vi "动态调用VI之间的数据.vi"() -> ()   [LabVIEW 2011]
panel:
  in  "Boolean":bool
  out "error IO":errorcluster
  out "signal type":T1(ring)
  out "frequency":dbl
  out "amplitude":dbl
  out "phase":dbl
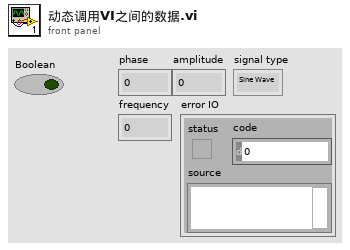
[diagram p1: front panel]
types:
  T1 = enum16{"Sine Wave", "Triangle Wave", "Square Wave", "Sawtooth Wave"}
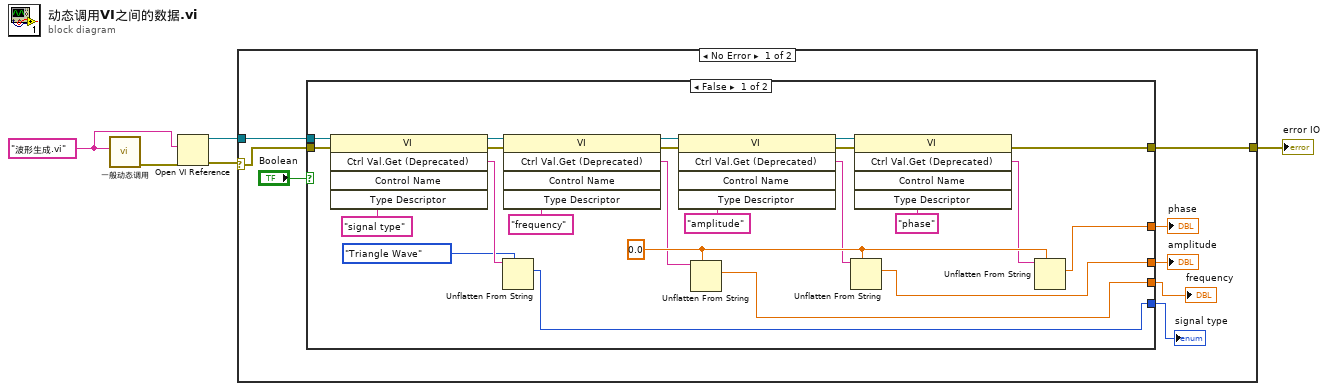
[diagram p0: block diagram]
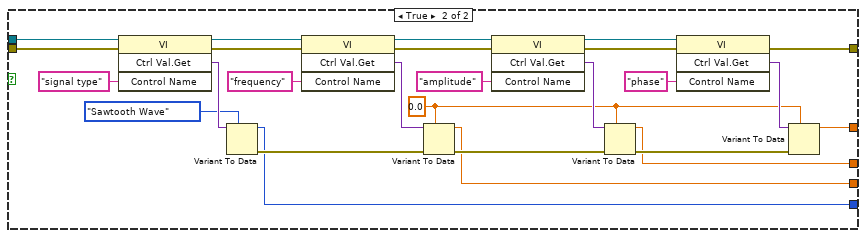
[diagram p2: hidden frame]
diagram:
  w4 = "波形生成.vi" ("name or relative path")
  n1 = call "一般动态调用.vi"("name or relative path"=w4) -> ("error out"=w5:errorcluster)  [unwired: 10 in]
  n2 = Open VI Reference(vi path=w4, error in (no error)=w5) -> (vi reference=w3:refnum<vi>, error out=w2:errorcluster)  [unwired: 4 in]
  n3 = case shown="No Error" w2 {
    selector: w2 -> [w12 w63]
    tunnel: w3 -> [w13 _]
    tunnel: [w7 w63] -> w1
    frame No Error {
      n4 = case shown="False" "Boolean" {
        tunnel: w13 -> [w36 w62]
        tunnel: w12 -> [w35 w61]
        tunnel: [w18 w41] -> w11
        tunnel: [w17 w40] -> w10
        tunnel: [w16 w39] -> w9
        tunnel: [w15 w38] -> w8
        tunnel: [w14 w37] -> w7
        frame False {
          w26 = 0.0 ("phase")
          n5 = invoke class="VI" method="Ctrl Val.Get (Deprecated)"(reference=w36, error in=w35, "Control Name"="signal type" ("控件名")) -> (reference out=w31:refnum<vi>, error out=w30:errorcluster, "Get Control Value"=w33:string)  [unwired: 2 in, 2 out]
          n6 = Unflatten From String(type=T1."Triangle Wave" ("signal type"), binary string=w33) -> (value=w15:T1)  [unwired: 3 in, 2 out]
          n7 = invoke class="VI" method="Ctrl Val.Get (Deprecated)"(reference=w31, error in=w30, "Control Name"="frequency" ("控件名")) -> (reference out=w25:refnum<vi>, error out=w24:errorcluster, "Get Control Value"=w21:string)  [unwired: 2 in, 2 out]
          n8 = invoke class="VI" method="Ctrl Val.Get (Deprecated)"(reference=w25, error in=w24, "Control Name"="amplitude" ("控件名")) -> (reference out=w23:refnum<vi>, error out=w22:errorcluster, "Get Control Value"=w20:string)  [unwired: 2 in, 2 out]
          n9 = Unflatten From String(type=w26, binary string=w21) -> (value=w16:dbl)  [unwired: 3 in, 2 out]
          n10 = Unflatten From String(type=w26, binary string=w20) -> (value=w17:dbl)  [unwired: 3 in, 2 out]
          n11 = invoke class="VI" method="Ctrl Val.Get (Deprecated)"(reference=w23, error in=w22, "Control Name"="phase" ("控件名")) -> (error out=w14:errorcluster, "Get Control Value"=w19:string)  [unwired: 2 in, 3 out]
          n12 = Unflatten From String(type=w26, binary string=w19) -> (value=w18:dbl)  [unwired: 3 in, 2 out]
        }
        frame True {
          w42 = 0.0
          n13 = invoke class="VI" method="Ctrl Val.Get"(reference=w62, error in=w61, "Control Name"="signal type") -> (reference out=w60:refnum<vi>, error out=w59:errorcluster, "Get Control Value Variant"=w58:variant)  [unwired: 1 in, 1 out]
          n14 = Variant To Data(type=T1."Sawtooth Wave", Variant=w58) -> (data=w38:T1, error out=w55:errorcluster)  [unwired: 1 in]
          n15 = invoke class="VI" method="Ctrl Val.Get"(reference=w60, error in=w59, "Control Name"="frequency") -> (reference out=w51:refnum<vi>, error out=w50:errorcluster, "Get Control Value Variant"=w54:variant)  [unwired: 1 in, 1 out]
          n16 = Variant To Data(error in=w55, type=w42, Variant=w54) -> (data=w39:dbl, error out=w48:errorcluster)
          n17 = invoke class="VI" method="Ctrl Val.Get"(reference=w51, error in=w50, "Control Name"="amplitude") -> (reference out=w47:refnum<vi>, error out=w46:errorcluster, "Get Control Value Variant"=w52:variant)  [unwired: 1 in, 1 out]
          n18 = Variant To Data(error in=w48, type=w42, Variant=w52) -> (data=w40:dbl, error out=w43:errorcluster)
          n19 = invoke class="VI" method="Ctrl Val.Get"(reference=w47, error in=w46, "Control Name"="phase") -> (error out=w37:errorcluster, "Get Control Value Variant"=w44:variant)  [unwired: 1 in, 2 out]
          n20 = Variant To Data(error in=w43, type=w42, Variant=w44) -> (data=w41:dbl)  [unwired: 1 out]
        }
      }
      "phase" <- w11
      "amplitude" <- w10
      "frequency" <- w9
      "signal type" <- w8
    }
    frame Error {
    }
  }
  "error IO" <- w1
